vi "SyncArrayCreator.vi"(9 "Sync2":bool, 10 "Sync1":bool, 11 "Sync0":bool) -> (3 "Array":bool[](array[boolean]))   [LabVIEW 2012]
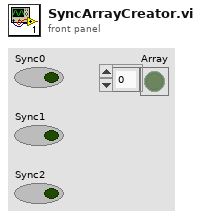
[diagram p1: front panel]
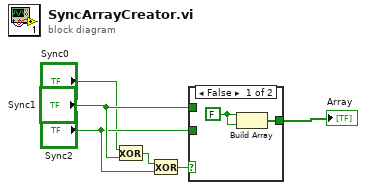
[diagram p0: block diagram]
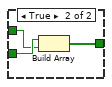
[diagram p2: hidden frame]
diagram:
  n1 = Exclusive Or(1:"Sync1", 2:"Sync0") -> (0:w1:bool)
  n2 = Exclusive Or(1:"Sync2", 2:w1) -> (0:w3:bool)
  n3 = case shown="False" w3 {
    tunnel: "Sync2" -> [_ w11]
    tunnel: "Sync1" -> [_ w10]
    tunnel: [w8 w9] -> w6
    frame False {
      w7 = FALSE ("Sync2 0A")
      n4 = Build Array(w7, w7) -> (w8:bool[])
    }
    frame True {
      n5 = Build Array(w11, w10) -> (w9:bool[])
    }
  }
  "Array" <- w6
